vi "Create Stabilizing Graph.vi"(10 "output cluster":T1, 11 "WaveformChart in":refnum<vi>) -> (3 "WaveformChart out":refnum<vi>)   [LabVIEW 2016]
uses:
  Controls/Cal Refs.ctl
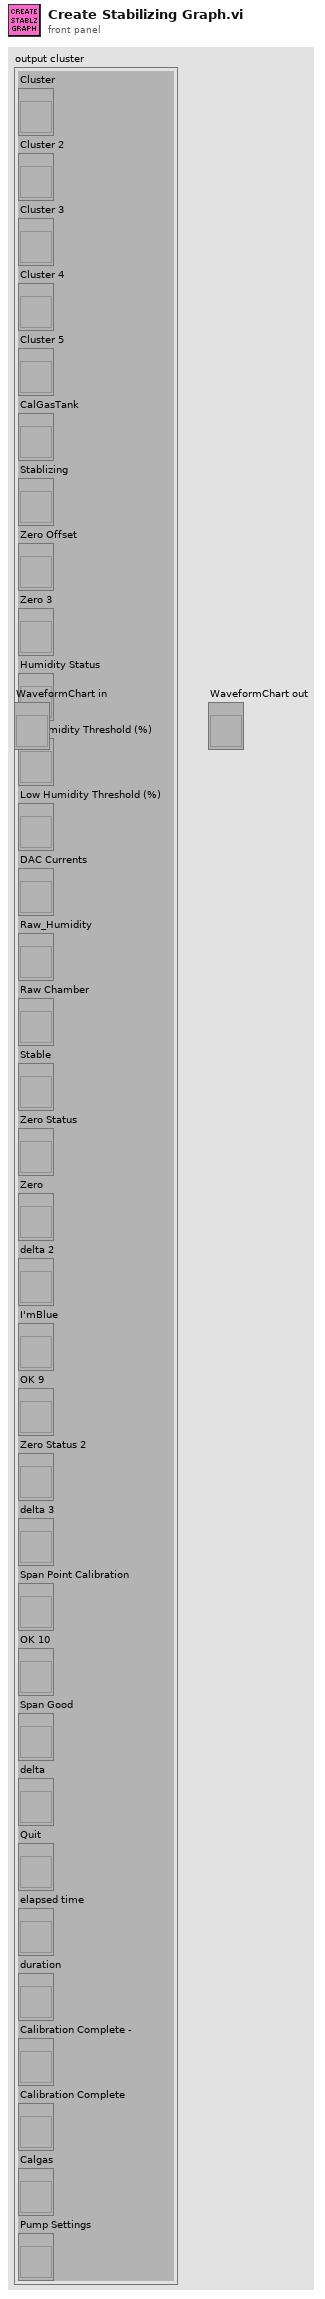
[diagram p1: front panel]
types:
  T1 = typedef "Cal Refs.ctl" = cluster{"Cluster":refnum<vi>, "Cluster 2":refnum<vi>, "Cluster 3":refnum<vi>, "Cluster 4":refnum<vi>, "Cluster 5":refnum<vi>, "CalGasTank":refnum<vi>, "Stablizing":refnum<vi>, "Zero Offset":refnum<vi>, "Zero 3":refnum<vi>, "Humidity Status":refnum<vi>, "Hi Humidity Threshold (%)":refnum<vi>, "Low Humidity Threshold (%)":refnum<vi>, "DAC Currents":refnum<vi>, "Raw_Humidity":refnum<vi>, "Raw Chamber":refnum<vi>, "Stable":refnum<vi>, "Zero Status":refnum<vi>, "Zero":refnum<vi>, "delta 2":refnum<vi>, "I'mBlue":refnum<vi>, "OK 9":refnum<vi>, "Zero Status 2":refnum<vi>, "delta 3":refnum<vi>, "Span Point Calibration":refnum<vi>, "OK 10":refnum<vi>, "Span Good":refnum<vi>, "delta":refnum<vi>, "Quit":refnum<vi>, "elapsed time":refnum<vi>, "duration":refnum<vi>, "Calibration Complete -":refnum<vi>, "Calibration Complete":refnum<vi>, "Calgas":refnum<vi>, "Pump Settings":refnum<vi>}
  T2 = cluster{"Tcal_Chamber":dbl, "Tcal_PCB":dbl, "Tcal_Film":dbl, "Tcal_Humidity":dbl, "Tcal_Det":dbl[], "Cal Gas":dbl, "Reference":dbl}
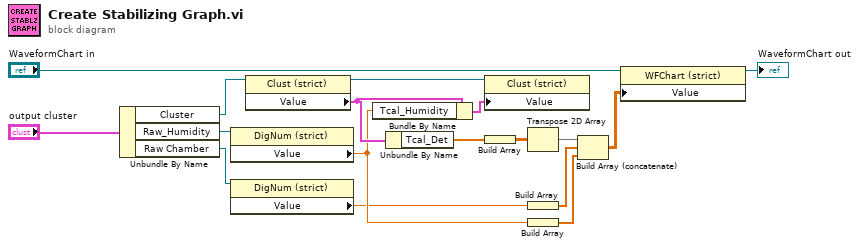
[diagram p0: block diagram]
diagram:
  n1 = Unbundle By Name("output cluster") -> ("Cluster"=w15:refnum<vi>, "Raw_Humidity"=w16:refnum<vi>, "Raw Chamber"=w17:refnum<vi>)
  n2 = property class="DigNum (strict)"(reference=w16) -> ("Value"=w5:dbl)  [unwired: 1 in, 2 out]
  n3 = property class="DigNum (strict)"(reference=w17) -> ("Value"=w3:dbl)  [unwired: 1 in, 2 out]
  n4 = property class="Clust (strict)"(reference=w15) -> (reference out=w4:refnum<vi>, "Value"=w9:T2)  [unwired: 1 in, 1 out]
  n5 = Bundle By Name(cluster=w9, "Tcal_Humidity"=w5) -> (w6:T2)
  n6 = Unbundle By Name(w9) -> ("Tcal_Det"=w8:dbl[])
  n7 = property class="Clust (strict)"(reference=w4, "Value"=w6) -> ()  [unwired: 1 in, 2 out]
  n8 = Build Array(w8) -> (w7:dbl[][])
  n9 = Transpose 2D Array(2D array=w7) -> (transposed array=w10:dbl[][])
  n10 = Build Array(w3) -> (w2:dbl[])
  n11 = Build Array(w5) -> (w1:dbl[])
  n12 = Build Array (concatenate)(w10, w2, w1) -> (w12:dbl[][])
  n13 = property on="Property Node" class="WFChart (strict)"(reference="WaveformChart in", "Value"=w12) -> (reference out=→"WaveformChart out":refnum<vi>)  [unwired: 1 in, 1 out]
